vi "gd_source_builder.vi"(7 "GD":bool) -> (2 "Gd switches":string)   [LabVIEW 2020]
uses:
  <vilib>/Utility/file.llb/Read Delimited Spreadsheet (string).vi
panel:
  in  "Diretório de trabalho":path=path "C:/ATP/ATPDraw/Projects_Flavio"
  in  "Lista de condições (arquivo.txt) 2":string="GDs.txt"
  out "GDs nodes":string[](array[string])
  # "CONSTROI SOURCE DA GD"
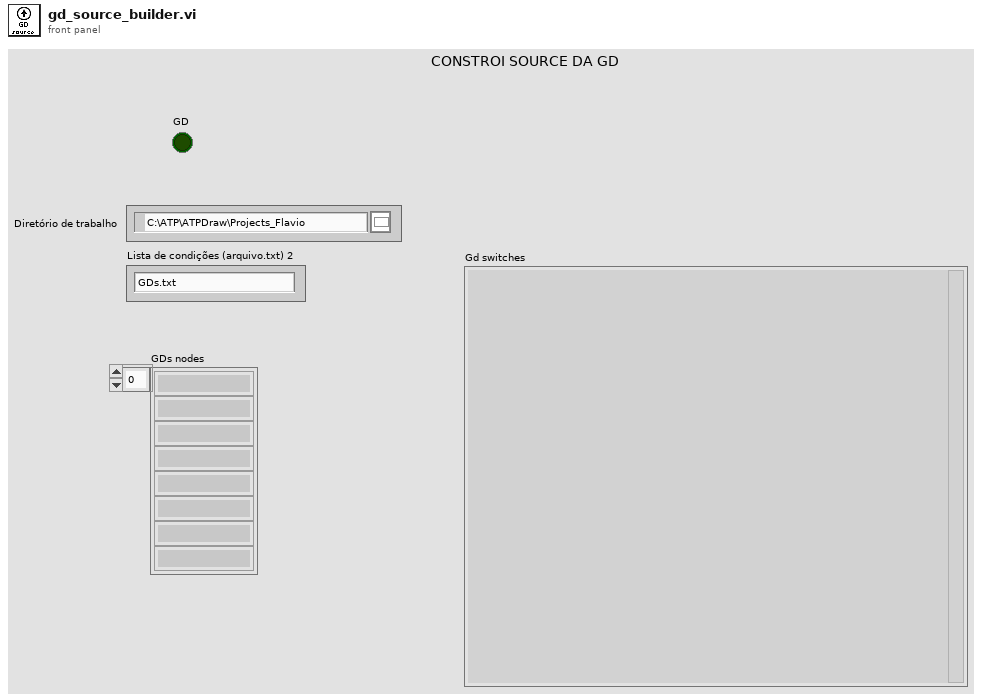
[diagram p1: front panel]
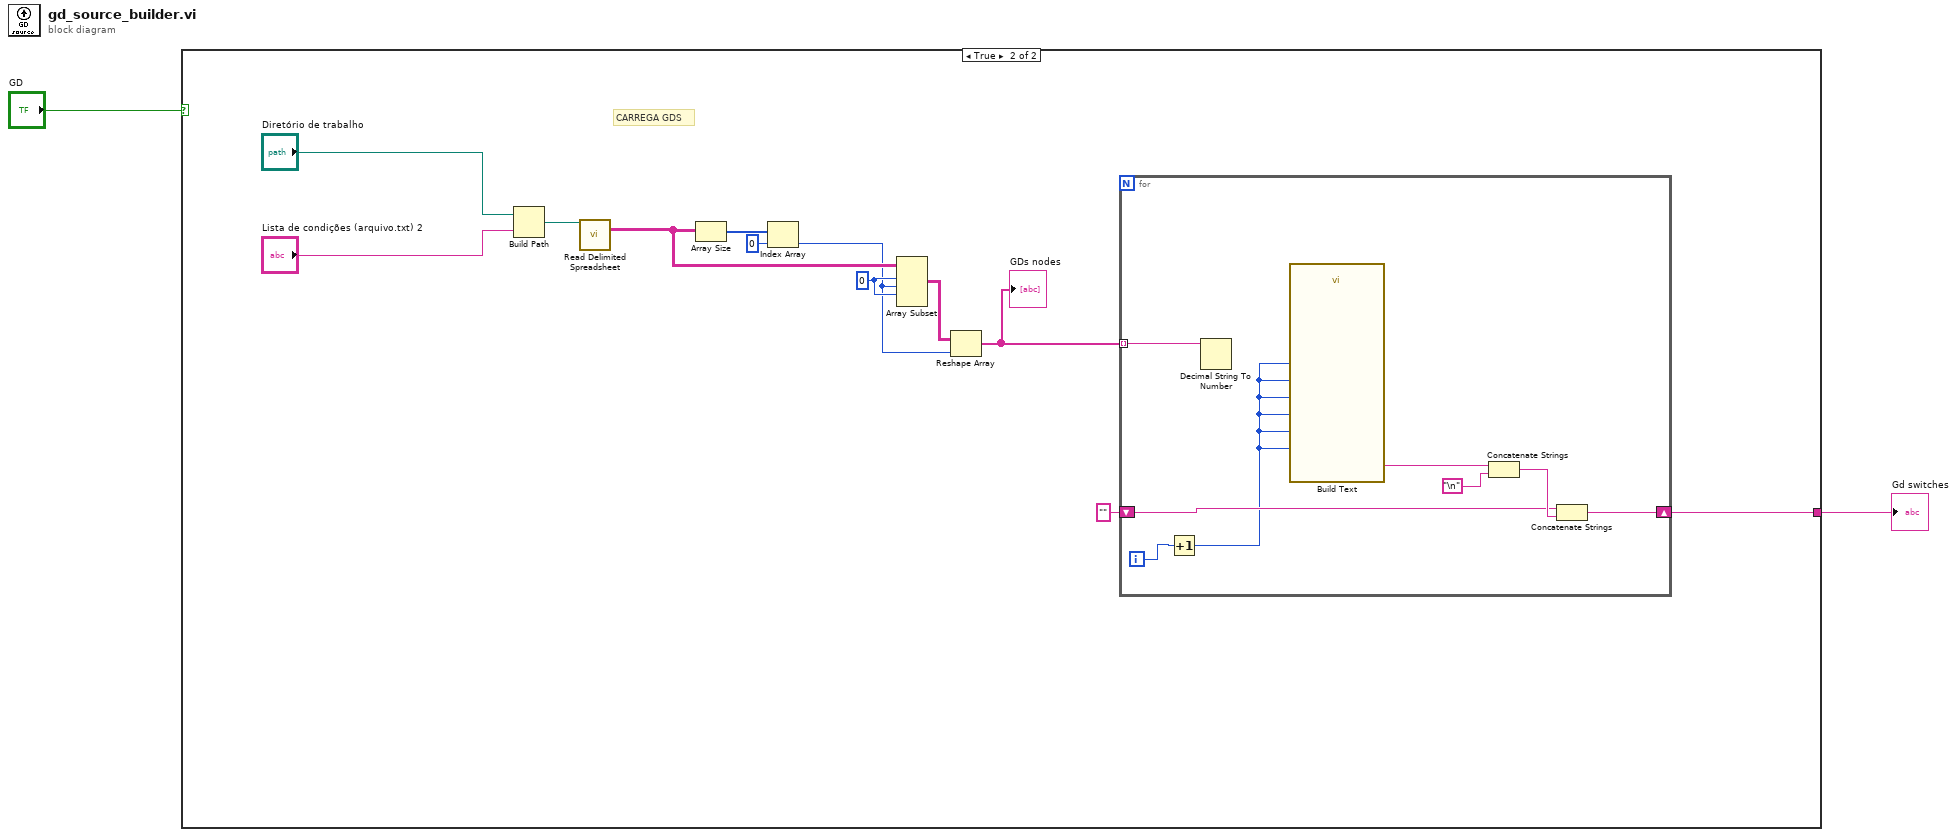
[diagram p0: block diagram]
diagram:
  n1 = case shown="True" "GD" {
    tunnel: [_ w4] -> w1
    frame False {
    }
    frame True {
      w12 = 0 ("index")
      # "CARREGA GDS"
      n2 = Build Path(base path="Diretório de trabalho", name or relative path="Lista de condições (arquivo.txt) 2") -> (appended path=w14:path)
      n3 = call-poly <vilib>:"Read Delimited Spreadsheet.vi"("file path (dialog if empty)"=w14) -> ("all rows"=w11:string[][])  [unwired: 9 in, 5 out]
      n4 = Array Size(array=w11) -> (size(s)=w10:i32[])
      n5 = Index Array(array=w10, index=0) -> (element=w6:i32)
      n6 = Array Subset(array=w11, index (row)=w12, length (row)=w6, index (col)=w12) -> (w8:string[][])  [unwired: 1 in]
      n7 = Reshape Array(w8, w6) -> (w5:string[])
      "GDs nodes" <- w5
      n8 = for {
        tunnel: w5 -> [w22] mode=indexing
        shift-right: [w17] -> w4
        shift-left: "" -> [w16]
        i -> [w21]
        n9 = Increment(x=w21) -> (x+1=w15:i32)
        n10 = Decimal String To Number(string=w22) -> ()  [unwired: 2 in, 2 out]
        n11 = call "Build Text"("Vg_c"=w15, "Vg_a"=w15, "Ig_a"=w15, "Ig_b"=w15, "Ig_c"=w15, "Vg_b"=w15) -> ("Result"=w18:string)  [unwired: 8 in, 1 out]
        n12 = Concatenate Strings(w18, "\n") -> (w19:string)
        n13 = Concatenate Strings(w16, w19) -> (w17:string)
      }
    }
  }
  "Gd switches" <- w1
